vi "PinholesRolling.vi"(4 "Current Threshold [nA]":dbl, 5 "settling\ndelay":i32) -> (1 "excluded channels":i32[](array[numeric]), 2 "Current [nA]":dbl[](array[numeric]), 3 "Flag":i32[](array[numeric]))   [LabVIEW 2019]
uses:
  general_VIs/globals/QC_MeasurementSetup.vi
  InstrControl/Switching/Switching.lvclass
  InstrControl/SupplyControl/SupplyControl.lvclass
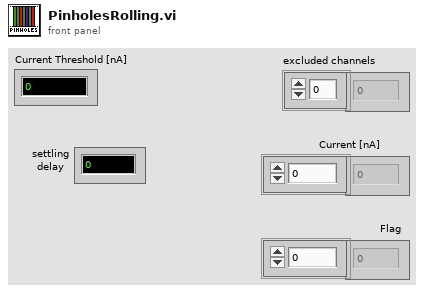
[diagram p1: front panel]
types:
  T1 = enum16{"Reference measurement", "Baseline correcetion 10V", "Baseline correcetion 100V", "Nothing"}
  T2 = cluster{"Bias Supply":refnum<class "SupplyControl.lvclass">, "SMU":refnum<class "SupplyControl.lvclass">, "LCR":refnum<class "LCRControl.lvclass">, "Probe Card Channels":i32, "Bias Voltage [V]":dbl, "First strip":i32, "Last strip":i32, "Base Voltage [V]":dbl, "Base Ramp Step [V]":dbl, "Base Ramp Interval [ms]":u32, "High Voltage [V]":dbl, "High Ramp Step [V]":dbl, "High Ramp Interval [ms]":u32, "AC frequency [Hz]":i32, "AC amplitude [V]":dbl, "RC Configuration":u16, "Single Needle":bool, "Temperature Readout":enum16{"Read Arduino", "Enter manually"}, "Arduino":refnum<class "ArduinoControl.lvclass">, "Fraction of good strips [%]":dbl, "ProbeStation":refnum<class "ProbeStationControl.lvclass">, "Switching":refnum<class "Switching.lvclass">, "Matrix used?":bool, "Matrix X Channels":cluster{"Bias Supply / SMU LO":i32, "Bias Supply / SMU HI":i32, "CV Box LO":i32, "CV Box HI":i32, "CV Box LO IN":i32, "CV Box HI IN":i32, "Volt meter LO":i32, "Volt meter HI":i32, "Mux1 C1":i32, "Mux1 C2":i32, "Mux2 C1":i32, "Mux2 C2":i32}, "Pinholes Y/N":bool, "Capacitance Y/N":bool, "Resistance Y/N":bool, "Bias Supply Name":string, "SMU Name":string, "LCR Name":string}
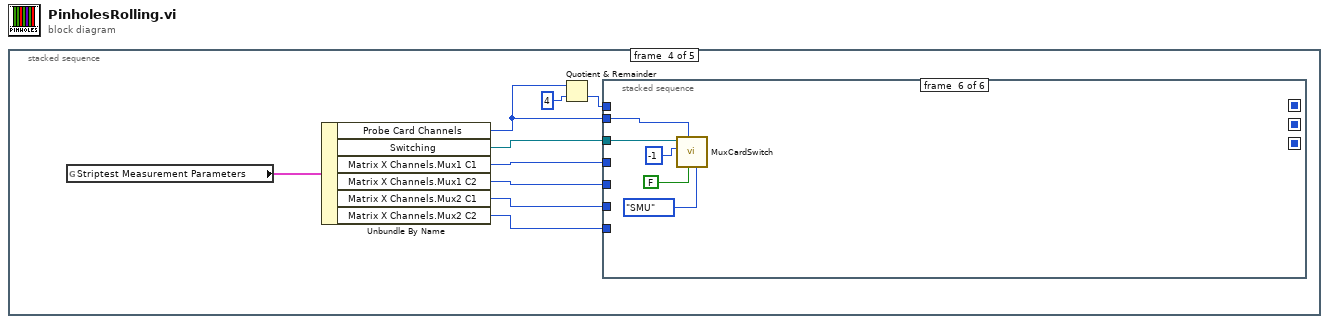
[diagram p0: block diagram]
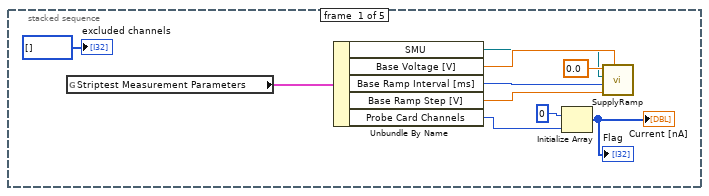
[diagram p2: hidden frame]
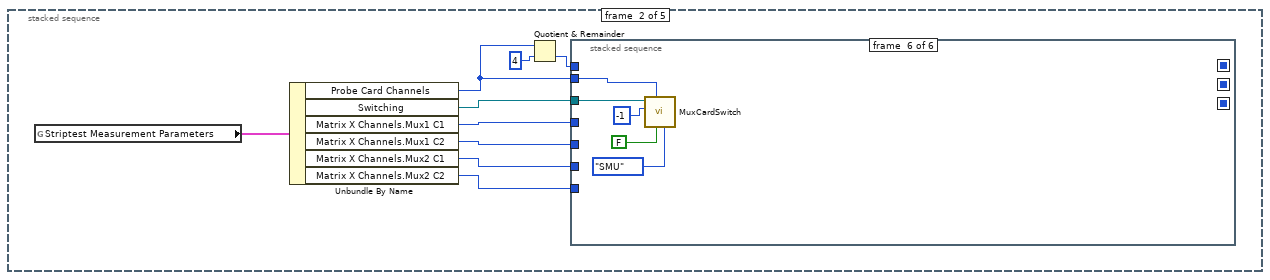
[diagram p3: hidden frame]
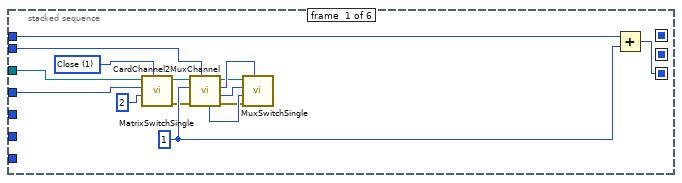
[diagram p4: hidden frame]
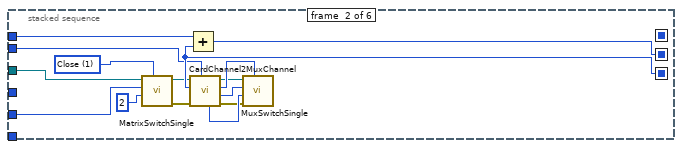
[diagram p5: hidden frame]
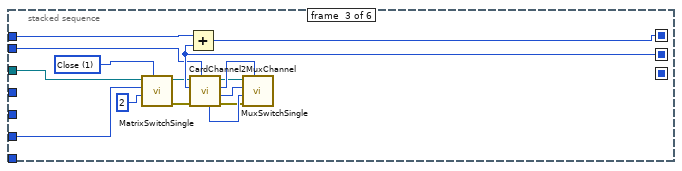
[diagram p6: hidden frame]
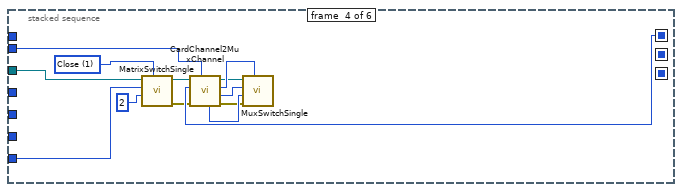
[diagram p7: hidden frame]
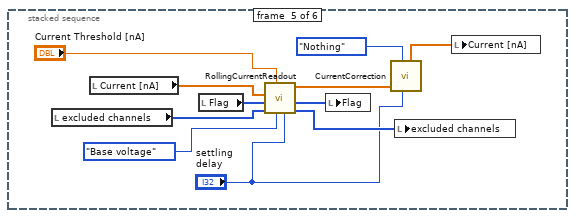
[diagram p8: hidden frame]
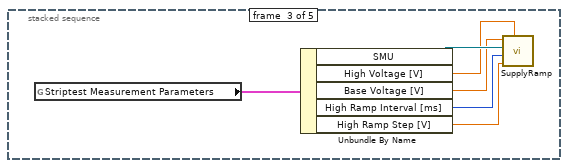
[diagram p9: hidden frame]
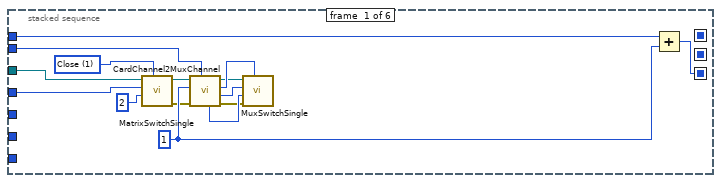
[diagram p10: hidden frame]
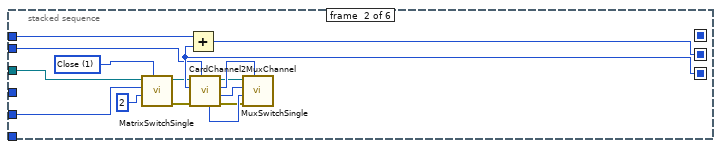
[diagram p11: hidden frame]
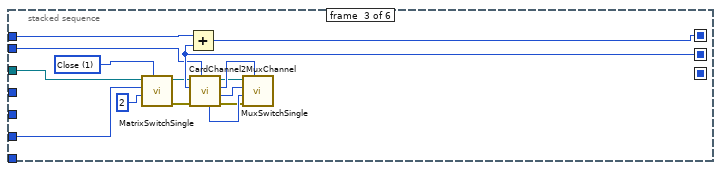
[diagram p12: hidden frame]
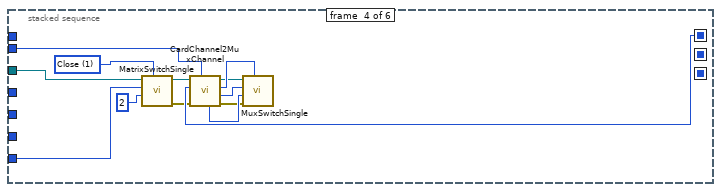
[diagram p13: hidden frame]
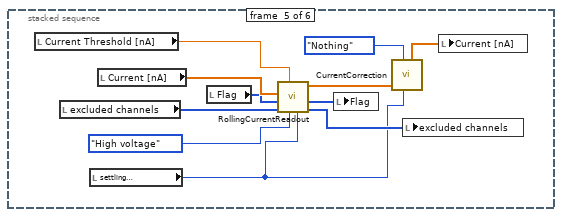
[diagram p14: hidden frame]
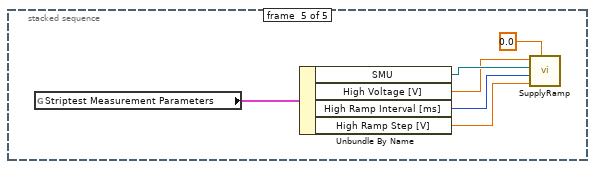
[diagram p15: hidden frame]
diagram:
  n1 = stacked-sequence {
    frame #0 {
      n2 = global read "QC_MeasurementSetup.vi" "Striptest Measurement Parameters"() -> (w6:T2)
      n3 = Unbundle By Name(w6) -> ("SMU"=w2:refnum<class "SupplyControl.lvclass">, "Base Voltage [V]"=w5:dbl, "Base Ramp Interval [ms]"=w4:u32, "Base Ramp Step [V]"=w3:dbl, "Probe Card Channels"=w1:i32)
      n4 = Initialize Array(0, w1) -> (→"Flag" →"Current [nA]":i32[])
      n5 = call "SupplyRamp.vi"("Requested Voltage"=w5, "Step Size"=w3, "Step Delay"=w4, "Supply IN"=w2, "Starting Voltage"=0.0) -> ()  [unwired: 3 in, 4 out]
      "excluded channels" <- i32[] []
    }
    frame #1 {
      n6 = global read "QC_MeasurementSetup.vi" "Striptest Measurement Parameters"() -> (w12:T2)
      n7 = Unbundle By Name(w12) -> ("Probe Card Channels"=w11:i32, "Switching"=w13:refnum<class "Switching.lvclass">, "Matrix X Channels.Mux1 C1"=w17:i32, "Matrix X Channels.Mux1 C2"=w16:i32, "Matrix X Channels.Mux2 C1"=w15:i32, "Matrix X Channels.Mux2 C2"=w14:i32)
      n8 = Quotient & Remainder(x=w11, y=4) -> (floor(x/y)=w18:i32)  [unwired: 1 out]
      n9 = stacked-sequence {
        seq-local: [w27 _ _ _ _ _] -> [_ w44 _ _ _ _]
        seq-local: [_ w43 _ _ _ _] -> [_ _ w58 _ _ _]
        seq-local: [_ _ w59 _ _ _] -> [_ _ _ w72 _ _]
        tunnel: w18 -> [w28 w36 w51 _ _ _]
        tunnel: w17 -> [w26 _ _ _ _ _]
        tunnel: w13 -> [w25 w37 w52 w66 _ w92]
        tunnel: w16 -> [_ w42 _ _ _ _]
        tunnel: w15 -> [_ _ w57 _ _ _]
        tunnel: w14 -> [_ _ _ w71 _ _]
        tunnel: w11 -> [w20 w35 w50 w65 _ w91]
        frame #0 {
          w29 = 1
          w34 = u16 1 items=["Open", "Close"] ("Switch action")
          n10 = call-dynamic "MatrixSwitchSingle.vi"("Switch action"=w34, "Matrix Y"=2, "Matrix X"=w26, "Switching in"=w25) -> ("error out"=w23:errorcluster, "Switching out"=w21:refnum<class "Switching.lvclass">)  [unwired: 5 in, 1 out]
          n11 = call-dynamic "CardChannel2MuxChannel.vi"("Probe Card Channels"=w20, "error in (no error)"=w23, "Probecard Channel No."=w29, "Switching in"=w21) -> ("error out"=w24:errorcluster, "C1 / C2"=w32:i32, "Mux No.:"=w31:u32, "Switching out"=w22:refnum<class "Switching.lvclass">, "Channel"=w33:i32)  [unwired: 2 in, 1 out]
          n12 = call-dynamic "MuxSwitchSingle.vi"("MUX address"=w31, "error in (no error)"=w24, "Channel"=w33, "C1 / C2"=w32, "Switching in"=w22) -> ()  [unwired: 4 in, 3 out]
          n13 = Add(x=w28, y=w29) -> (x+y=w27:i32)
        }
        frame #1 {
          w46 = u16 1 items=["Open", "Close"] ("Switch action")
          n14 = call-dynamic "MatrixSwitchSingle.vi"("Switch action"=w46, "Matrix Y"=2, "Matrix X"=w42, "Switching in"=w37) -> ("error out"=w39:errorcluster, "Switching out"=w38:refnum<class "Switching.lvclass">)  [unwired: 5 in, 1 out]
          n15 = Add(x=w36, y=w44) -> (x+y=w43:i32)
          n16 = call-dynamic "CardChannel2MuxChannel.vi"("Probe Card Channels"=w35, "error in (no error)"=w39, "Probecard Channel No."=w44, "Switching in"=w38) -> ("error out"=w40:errorcluster, "C1 / C2"=w48:i32, "Mux No.:"=w47:u32, "Switching out"=w41:refnum<class "Switching.lvclass">, "Channel"=w49:i32)  [unwired: 2 in, 1 out]
          n17 = call-dynamic "MuxSwitchSingle.vi"("MUX address"=w47, "error in (no error)"=w40, "Channel"=w49, "C1 / C2"=w48, "Switching in"=w41) -> ()  [unwired: 4 in, 3 out]
        }
        frame #2 {
          w63 = u16 1 items=["Open", "Close"] ("Switch action")
          n18 = call-dynamic "MatrixSwitchSingle.vi"("Switch action"=w63, "Matrix Y"=2, "Matrix X"=w57, "Switching in"=w52) -> ("error out"=w56:errorcluster, "Switching out"=w55:refnum<class "Switching.lvclass">)  [unwired: 5 in, 1 out]
          n19 = Add(x=w51, y=w58) -> (x+y=w59:i32)
          n20 = call-dynamic "CardChannel2MuxChannel.vi"("Probe Card Channels"=w50, "error in (no error)"=w56, "Probecard Channel No."=w58, "Switching in"=w55) -> ("error out"=w53:errorcluster, "C1 / C2"=w61:i32, "Mux No.:"=w62:u32, "Switching out"=w54:refnum<class "Switching.lvclass">, "Channel"=w60:i32)  [unwired: 2 in, 1 out]
          n21 = call-dynamic "MuxSwitchSingle.vi"("MUX address"=w62, "error in (no error)"=w53, "Channel"=w60, "C1 / C2"=w61, "Switching in"=w54) -> ()  [unwired: 4 in, 3 out]
        }
        frame #3 {
          w74 = u16 1 items=["Open", "Close"] ("Switch action")
          n22 = call-dynamic "MatrixSwitchSingle.vi"("Switch action"=w74, "Matrix Y"=2, "Matrix X"=w71, "Switching in"=w66) -> ("error out"=w68:errorcluster, "Switching out"=w70:refnum<class "Switching.lvclass">)  [unwired: 5 in, 1 out]
          n23 = call-dynamic "CardChannel2MuxChannel.vi"("Probe Card Channels"=w65, "error in (no error)"=w68, "Probecard Channel No."=w72, "Switching in"=w70) -> ("error out"=w67:errorcluster, "C1 / C2"=w76:i32, "Mux No.:"=w75:u32, "Switching out"=w69:refnum<class "Switching.lvclass">, "Channel"=w77:i32)  [unwired: 2 in, 1 out]
          n24 = call-dynamic "MuxSwitchSingle.vi"("MUX address"=w75, "error in (no error)"=w67, "Channel"=w77, "C1 / C2"=w76, "Switching in"=w69) -> ()  [unwired: 4 in, 3 out]
        }
        frame #4 {
          n25 = local read "excluded channels"() -> (w86:i32[])
          n26 = local read "Current [nA]"() -> (w87:dbl[])
          n27 = local read "Flag"() -> (w85:i32[])
          n28 = call "RollingCurrentReadout.vi"("settling\ndelay"="settling\ndelay", "Base/High Voltage?"=enum16{"Base voltage", "High voltage"}."Base voltage", "Current Threshold [nA]"="Current Threshold [nA]", "disabled channels IN"=w86, "Flag IN"=w85, "Current Array IN [nA]"=w87) -> ("disabled channels OUT"=w84:i32[], "Flag OUT"=w83:i32[], "Current Array OUT [nA]"=w82:dbl[])  [unwired: 2 in, 1 out]
          n29 = local write "Flag"(w83) -> ()
          n30 = call "CurrentCorrection.vi"("Action"=T1."Nothing", "Current IN"=w82, "settling\ndelay"="settling\ndelay") -> ("Current OUT"=w81:dbl[])  [unwired: 2 in, 4 out]
          n31 = local write "excluded channels"(w84) -> ()
          n32 = local write "Current [nA]"(w81) -> ()
        }
        frame #5 {
          n33 = call-dynamic "MuxCardSwitch.vi"("Instrument"=enum16{"SMU", "LCR"}."SMU", "Single Needle"=FALSE, "Probe Card Channels"=w91, "Switch to channel"=-1, "Switching in"=w92) -> ()  [unwired: 4 in, 3 out]
        }
      }
    }
    frame #2 {
      n34 = global read "QC_MeasurementSetup.vi" "Striptest Measurement Parameters"() -> (w99:T2)
      n35 = Unbundle By Name(w99) -> ("SMU"=w96:refnum<class "SupplyControl.lvclass">, "High Voltage [V]"=w94:dbl, "Base Voltage [V]"=w95:dbl, "High Ramp Interval [ms]"=w97:u32, "High Ramp Step [V]"=w98:dbl)
      n36 = call "SupplyRamp.vi"("Requested Voltage"=w94, "Step Size"=w98, "Step Delay"=w97, "Supply IN"=w96, "Starting Voltage"=w95) -> ()  [unwired: 3 in, 4 out]
    }
    frame #3 {
      n37 = global read "QC_MeasurementSetup.vi" "Striptest Measurement Parameters"() -> (w101:T2)
      n38 = Unbundle By Name(w101) -> ("Probe Card Channels"=w100:i32, "Switching"=w106:refnum<class "Switching.lvclass">, "Matrix X Channels.Mux1 C1"=w105:i32, "Matrix X Channels.Mux1 C2"=w104:i32, "Matrix X Channels.Mux2 C1"=w103:i32, "Matrix X Channels.Mux2 C2"=w102:i32)
      n39 = Quotient & Remainder(x=w100, y=4) -> (floor(x/y)=w107:i32)  [unwired: 1 out]
      n40 = stacked-sequence {
        seq-local: [w116 _ _ _ _ _] -> [_ w133 _ _ _ _]
        seq-local: [_ w132 _ _ _ _] -> [_ _ w148 _ _ _]
        seq-local: [_ _ w147 _ _ _] -> [_ _ _ w161 _ _]
        tunnel: w107 -> [w118 w125 w140 _ _ _]
        tunnel: w106 -> [w115 w126 w141 w155 _ w180]
        tunnel: w105 -> [w114 _ _ _ _ _]
        tunnel: w100 -> [w109 w124 w139 w154 _ w179]
        tunnel: w104 -> [_ w131 _ _ _ _]
        tunnel: w103 -> [_ _ w146 _ _ _]
        tunnel: w102 -> [_ _ _ w160 _ _]
        frame #0 {
          w117 = 1
          w123 = u16 1 items=["Open", "Close"] ("Switch action")
          n41 = call-dynamic "MatrixSwitchSingle.vi"("Switch action"=w123, "Matrix Y"=2, "Matrix X"=w114, "Switching in"=w115) -> ("error out"=w111:errorcluster, "Switching out"=w113:refnum<class "Switching.lvclass">)  [unwired: 5 in, 1 out]
          n42 = call-dynamic "CardChannel2MuxChannel.vi"("Probe Card Channels"=w109, "error in (no error)"=w111, "Probecard Channel No."=w117, "Switching in"=w113) -> ("error out"=w110:errorcluster, "C1 / C2"=w121:i32, "Mux No.:"=w120:u32, "Switching out"=w112:refnum<class "Switching.lvclass">, "Channel"=w122:i32)  [unwired: 2 in, 1 out]
          n43 = call-dynamic "MuxSwitchSingle.vi"("MUX address"=w120, "error in (no error)"=w110, "Channel"=w122, "C1 / C2"=w121, "Switching in"=w112) -> ()  [unwired: 4 in, 3 out]
          n44 = Add(x=w118, y=w117) -> (x+y=w116:i32)
        }
        frame #1 {
          w135 = u16 1 items=["Open", "Close"] ("Switch action")
          n45 = call-dynamic "MatrixSwitchSingle.vi"("Switch action"=w135, "Matrix Y"=2, "Matrix X"=w131, "Switching in"=w126) -> ("error out"=w130:errorcluster, "Switching out"=w129:refnum<class "Switching.lvclass">)  [unwired: 5 in, 1 out]
          n46 = Add(x=w125, y=w133) -> (x+y=w132:i32)
          n47 = call-dynamic "CardChannel2MuxChannel.vi"("Probe Card Channels"=w124, "error in (no error)"=w130, "Probecard Channel No."=w133, "Switching in"=w129) -> ("error out"=w128:errorcluster, "C1 / C2"=w137:i32, "Mux No.:"=w136:u32, "Switching out"=w127:refnum<class "Switching.lvclass">, "Channel"=w138:i32)  [unwired: 2 in, 1 out]
          n48 = call-dynamic "MuxSwitchSingle.vi"("MUX address"=w136, "error in (no error)"=w128, "Channel"=w138, "C1 / C2"=w137, "Switching in"=w127) -> ()  [unwired: 4 in, 3 out]
        }
        frame #2 {
          w152 = u16 1 items=["Open", "Close"] ("Switch action")
          n49 = call-dynamic "MatrixSwitchSingle.vi"("Switch action"=w152, "Matrix Y"=2, "Matrix X"=w146, "Switching in"=w141) -> ("error out"=w145:errorcluster, "Switching out"=w142:refnum<class "Switching.lvclass">)  [unwired: 5 in, 1 out]
          n50 = Add(x=w140, y=w148) -> (x+y=w147:i32)
          n51 = call-dynamic "CardChannel2MuxChannel.vi"("Probe Card Channels"=w139, "error in (no error)"=w145, "Probecard Channel No."=w148, "Switching in"=w142) -> ("error out"=w144:errorcluster, "C1 / C2"=w150:i32, "Mux No.:"=w151:u32, "Switching out"=w143:refnum<class "Switching.lvclass">, "Channel"=w149:i32)  [unwired: 2 in, 1 out]
          n52 = call-dynamic "MuxSwitchSingle.vi"("MUX address"=w151, "error in (no error)"=w144, "Channel"=w149, "C1 / C2"=w150, "Switching in"=w143) -> ()  [unwired: 4 in, 3 out]
        }
        frame #3 {
          w163 = u16 1 items=["Open", "Close"] ("Switch action")
          n53 = call-dynamic "MatrixSwitchSingle.vi"("Switch action"=w163, "Matrix Y"=2, "Matrix X"=w160, "Switching in"=w155) -> ("error out"=w159:errorcluster, "Switching out"=w156:refnum<class "Switching.lvclass">)  [unwired: 5 in, 1 out]
          n54 = call-dynamic "CardChannel2MuxChannel.vi"("Probe Card Channels"=w154, "error in (no error)"=w159, "Probecard Channel No."=w161, "Switching in"=w156) -> ("error out"=w158:errorcluster, "C1 / C2"=w165:i32, "Mux No.:"=w164:u32, "Switching out"=w157:refnum<class "Switching.lvclass">, "Channel"=w166:i32)  [unwired: 2 in, 1 out]
          n55 = call-dynamic "MuxSwitchSingle.vi"("MUX address"=w164, "error in (no error)"=w158, "Channel"=w166, "C1 / C2"=w165, "Switching in"=w157) -> ()  [unwired: 4 in, 3 out]
        }
        frame #4 {
          n56 = local read "Current Threshold [nA]"() -> (w172:dbl)
          n57 = local read "excluded channels"() -> (w176:i32[])
          n58 = local read "settling\ndelay"() -> (w168:i32)
          n59 = local read "Current [nA]"() -> (w177:dbl[])
          n60 = local read "Flag"() -> (w175:i32[])
          n61 = call "RollingCurrentReadout.vi"("settling\ndelay"=w168, "Base/High Voltage?"=enum16{"Base voltage", "High voltage"}."High voltage", "Current Threshold [nA]"=w172, "disabled channels IN"=w176, "Flag IN"=w175, "Current Array IN [nA]"=w177) -> ("disabled channels OUT"=w174:i32[], "Flag OUT"=w173:i32[], "Current Array OUT [nA]"=w171:dbl[])  [unwired: 2 in, 1 out]
          n62 = local write "Flag"(w173) -> ()
          n63 = call "CurrentCorrection.vi"("Action"=T1."Nothing", "Current IN"=w171, "settling\ndelay"=w168) -> ("Current OUT"=w170:dbl[])  [unwired: 2 in, 4 out]
          n64 = local write "excluded channels"(w174) -> ()
          n65 = local write "Current [nA]"(w170) -> ()
        }
        frame #5 {
          n66 = call-dynamic "MuxCardSwitch.vi"("Instrument"=enum16{"SMU", "LCR"}."SMU", "Single Needle"=FALSE, "Probe Card Channels"=w179, "Switch to channel"=-1, "Switching in"=w180) -> ()  [unwired: 4 in, 3 out]
        }
      }
    }
    frame #4 {
      n67 = global read "QC_MeasurementSetup.vi" "Striptest Measurement Parameters"() -> (w187:T2)
      n68 = Unbundle By Name(w187) -> ("SMU"=w186:refnum<class "SupplyControl.lvclass">, "High Voltage [V]"=w183:dbl, "High Ramp Interval [ms]"=w184:u32, "High Ramp Step [V]"=w185:dbl)
      n69 = call "SupplyRamp.vi"("Requested Voltage"=0.0, "Step Size"=w185, "Step Delay"=w184, "Supply IN"=w186, "Starting Voltage"=w183) -> ()  [unwired: 3 in, 4 out]
    }
  }
